vi "SimpleCalc.vi"() -> ()   [LabVIEW 2020]
panel:
  in  "Ring":u16(ring) items=["DIV", "MUL", "SUB", "ADD"]
  out "Numeric 3":dbl
  in  "Numeric 2":dbl
  in  "Numeric":dbl
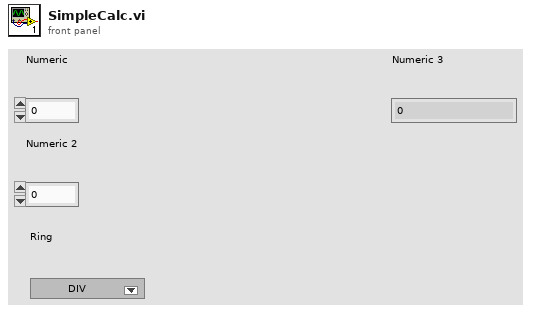
[diagram p1: front panel]
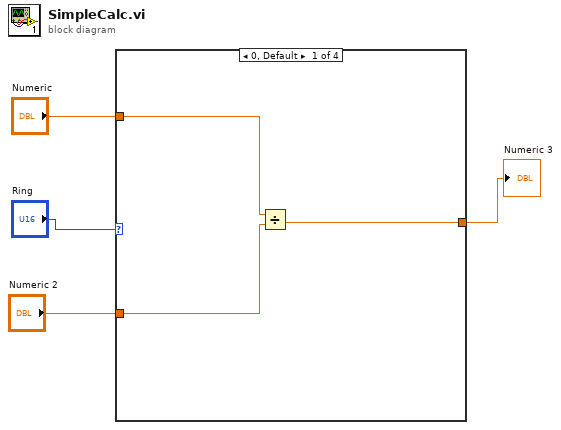
[diagram p0: block diagram]
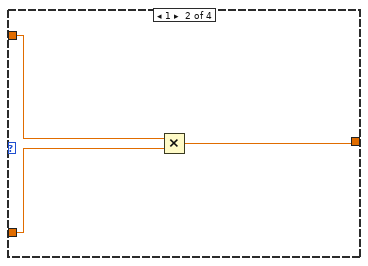
[diagram p2: hidden frame]
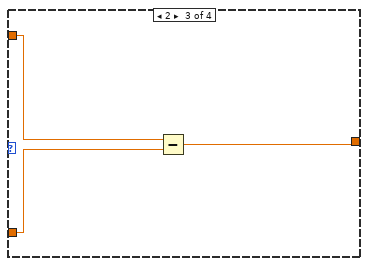
[diagram p3: hidden frame]
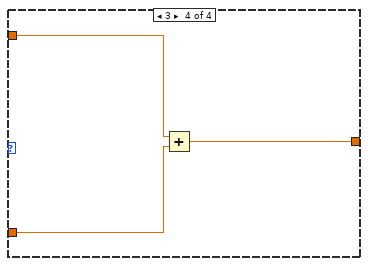
[diagram p4: hidden frame]
diagram:
  n1 = case shown="0, Default" "Ring" {
    tunnel: "Numeric" -> [w7 w10 w13 w16]
    tunnel: "Numeric 2" -> [w6 w9 w12 w15]
    tunnel: [w5 w8 w11 w14] -> w1
    frame 0, Default {
      n2 = Divide(x=w7, y=w6) -> (x/y=w5:dbl)
    }
    frame 1 {
      n3 = Multiply(x=w10, y=w9) -> (x*y=w8:dbl)
    }
    frame 2 {
      n4 = Subtract(x=w13, y=w12) -> (x-y=w11:dbl)
    }
    frame 3 {
      n5 = Add(x=w16, y=w15) -> (x+y=w14:dbl)
    }
  }
  "Numeric 3" <- w1
